vi "NumFreqs.vi"(7 "TestParams":dbl[][](array[numeric])) -> (3 "NumFreqs":i32)   [LabVIEW 2018, in "AnalysisPlugins.lvlib" / "PmuAnalysis.lvclass"]
uses:
  PmuAnalysis.lvclass
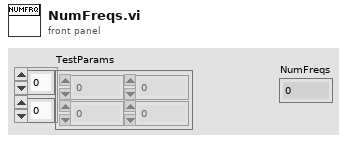
[diagram p1: front panel]
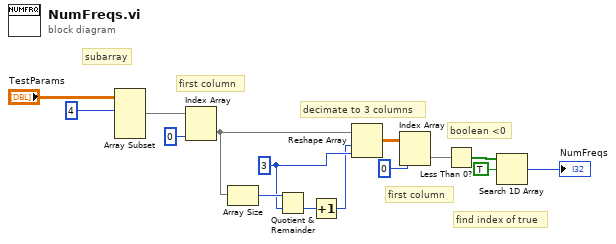
[diagram p0: block diagram]
diagram:
  w11 = 3 ("dimension size")
  # "find index of true"
  # "boolean <0"
  # "first column"
  # "decimate to 3 columns"
  # "first column"
  # "subarray"
  n1 = Array Subset(array="TestParams", index (row)=4 ("index")) -> (w3:dbl[][])  [unwired: 3 in]
  n2 = Index Array(array=w3, index (col)=0 ("disabled index (col)")) -> (element=w13:dbl[])  [unwired: 1 in]
  n3 = Array Size(array=w13) -> (size(s)=w12:i32)
  n4 = Quotient & Remainder(x=w12, y=w11) -> (floor(x/y)=w10:i32)  [unwired: 1 out]
  n5 = Increment(x=w10) -> (x+1=w9:i32)
  n6 = Reshape Array(w13, w9, w11) -> (w8:dbl[][])
  n7 = Index Array(array=w8, index (col)=0 ("disabled index (col)")) -> (element=w6:dbl[])  [unwired: 1 in]
  n8 = Less Than 0?(x=w6) -> (x < 0?=w5:bool[])
  n9 = Search 1D Array(1D array=w5, element=TRUE) -> (index of element=→"NumFreqs":i32)  [unwired: 1 in]
